vi "Sub Bytes.vi"(2 "Nb":i32=4, 7 "State In":u16[][](array[numeric])=[[125, 216, 135, 144], [71, 71, 164, 177], [128, 52, 170, 55], [161, 141, 234, 198]], 11 "error in":errorcluster) -> (8 "State Out":u16[][](array[numeric]), 15 "error out":errorcluster)   [LabVIEW 2020, in "Library Commun.lvlib" / "Advanced Encryption Standard (AES).lvlib"]
doc: "In the SubBytes step, each byte in the matrix is updated using an 8-bit substitution box, the Rijndael S-box. This operation provides the non-linearity in the cipher. \n\n<inline>"
uses:
  Advanced Encryption Standard (AES).lvlib
panel:
  # "old s= 125,216,135,144,71,71,164,177,128,52,170,55,161,141,234,198"
  # "new s= 255,97,23,96,160,160,73,200,205,24,172,154,50,93,135,180"
  # "255,97,23,96,160,73,200,160,172,154,205,24,        180,50,93,135"
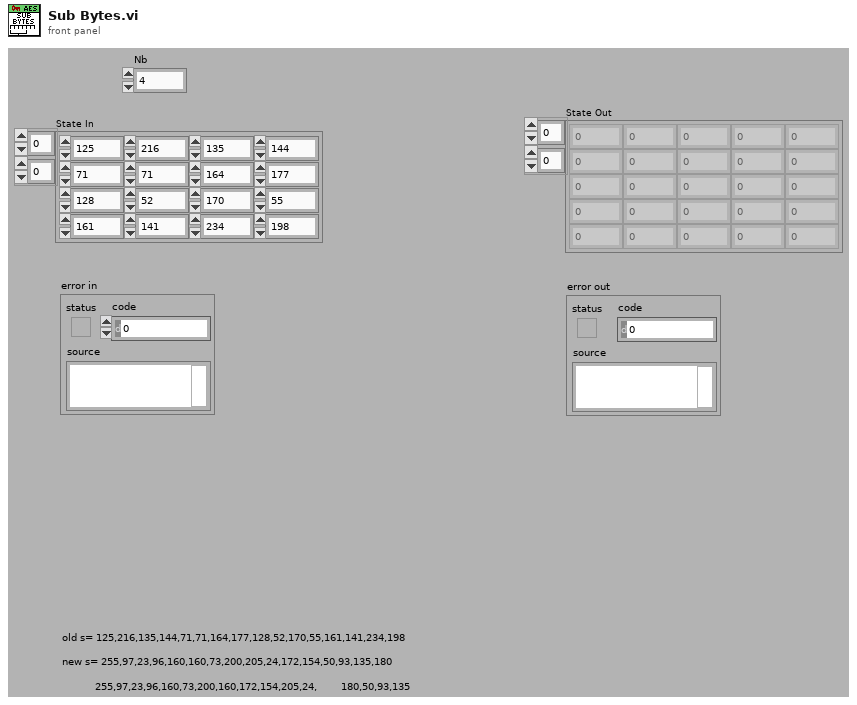
[diagram p1: front panel]
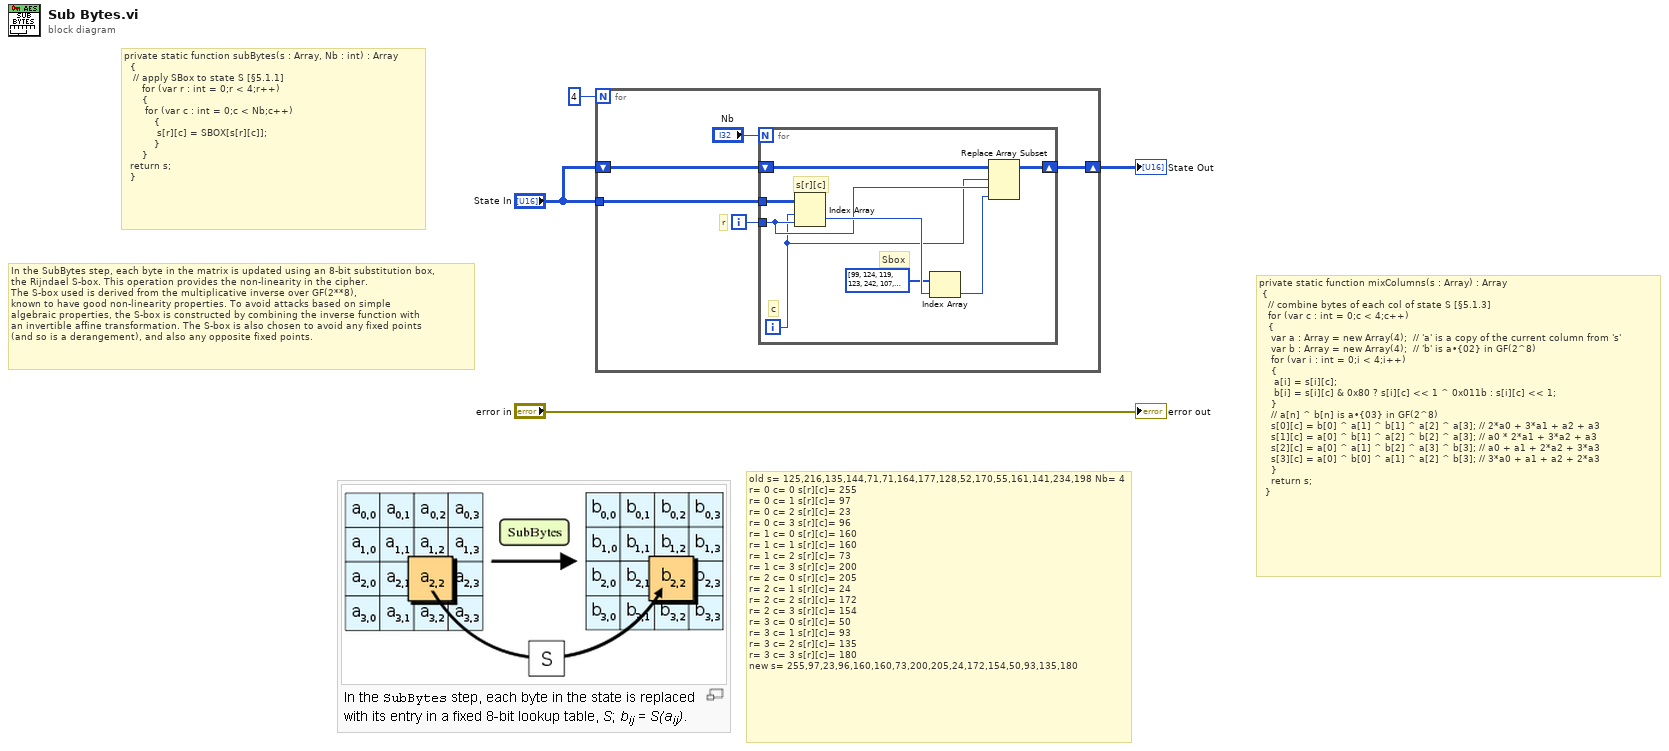
[diagram p0: block diagram]
diagram:
  # "In the SubBytes step, each byte in the matrix is updated using an 8-bit substitution box, \nthe Rijndael S-box. This operation provides the non-linearity in the cipher. \nThe S-box used is derived from the multiplicative inverse over GF(2**8), \nknown to have good non-linearity properties. To avoid attacks based on simple \nalgebraic properties, the S-box is constructed by combining the inverse function with \nan invertible affine transformation. The S-box is also chosen to avoid any fixed points \n(and so is a derangement), and also any opposite fixed points."
  # "old s= 125,216,135,144,71,71,164,177,128,52,170,55,161,141,234,198 Nb= 4\nr= 0 c= 0 s[r][c]= 255\nr= 0 c= 1 s[r][c]= 97\nr= 0 c= 2 s[r][c]= 23\nr= 0 c= 3 s[r][c]= 96\nr= 1 c= 0 s[r][c]= 160\nr= 1 c= 1 s[r][c]= 160\nr= 1 c= 2 s[r][c]= 73\nr= 1 c= 3 s[r][c]= 200\nr= 2 c= 0 s[r][c]= 205\nr= 2 c= 1 s[r][c]= 24\nr= 2 c= 2 s[r][c]= 172\nr= 2 c= 3 s[r][c]= 154\nr= 3 c= 0 s[r][c]= 50\nr= 3 c= 1 s[r][c]= 93\nr= 3 c= 2 s[r][c]= 135\nr= 3 c= 3 s[r][c]= 180\nnew s= 255,97,23,96,160,160,73,200,205,24,172,154,50,93,135,180"
  # "private static function subBytes(s : Array, Nb : int) : Array \n\t\t{    \n\t\t\t// apply SBox to state S [§5.1.1]\n\t\t   \tfor (var r : int = 0;r < 4;r++) \n\t\t   \t{\n\t\t   \t\tfor (var c : int = 0;c < Nb;c++) \n\t\t      \t\t{\n\t\t\t      \t\ts[r][c] = SBOX[s[r][c]];\n\t\t\t      \t}\n   \t\t\t}\n\t\treturn s;\t\t\t\n\t\t}"
  # "private static function mixColumns(s : Array) : Array \n {   \n\t\t\t// combine bytes of each col of state S [§5.1.3]\n\t\t\tfor (var c : int = 0;c < 4;c++) \n\t\t\t{\n\t\t\t\tvar a : Array = new Array(4);  // 'a' is a copy of the current column from 's'\n\t\t\t\tvar b : Array = new Array(4);  // 'b' is a•{02} in GF(2^8)\n\t\t\t\tfor (var i : int = 0;i < 4;i++) \n\t\t\t\t{\n\t\t\t\t\ta[i] = s[i][c];\n\t\t\t\t\tb[i] = s[i][c] & 0x80 ? s[i][c] << 1 ^ 0x011b : s[i][c] << 1;\n\t\t\t\t}\n\t\t\t\t// a[n] ^ b[n] is a•{03} in GF(2^8)\n\t\t\t\ts[0][c] = b[0] ^ a[1] ^ b[1] ^ a[2] ^ a[3]; // 2*a0 + 3*a1 + a2 + a3\n\t\t\t\ts[1][c] = a[0] ^ b[1] ^ a[2] ^ b[2] ^ a[3]; // a0 * 2*a1 + 3*a2 + a3\n\t\t\t\ts[2][c] = a[0] ^ a[1] ^ b[2] ^ a[3] ^ b[3]; // a0 + a1 + 2*a2 + 3*a3\n\t\t\t\ts[3][c] = a[0] ^ b[0] ^ a[1] ^ a[2] ^ b[3]; // 3*a0 + a1 + a2 + 2*a3\n\t\t\t\t}\n\t\t\t\treturn s;\n\t\t}"
  n1 = for {
    N: 4 -> [_]
    tunnel: "State In" -> [w8]
    shift-right: [w5] -> w2
    shift-left: "State In" -> [w7]
    i -> [w9]
    # "r"
    n2 = for {
      N: "Nb" -> [_]
      tunnel: w8 -> [w17]
      tunnel: w9 -> [w14]
      shift-right: [w10] -> w5
      shift-left: w7 -> [w11]
      i -> [w13]
      # "Sbox"
      # "s[r][c]"
      # "c"
      n3 = Index Array(array=w17, index (row)=w13, index (col)=w14) -> (element=w16:u16)
      n4 = Index Array(array=u16[] [99, 124, 119, 123, 242, 107, 111, 197, 48, 1, 103, 43, 254, 215, 171, 118, 202, 130, 201, 125, 250, 89, 71, 240, 173, 212, 162, 175, 156, 164, 114, 192, 183, 253, 147, 38, 54, 63, 247, 204, 52, 165, 229, 241, 113, 216, 49, 21, 4, 199, 35, 195, 24, 150, 5, 154, 7, 18, 128, 226, 235, 39, 178, 117, 9, 131, 44, 26, 27, 110, 90, 160, 82, 59, 214, 179, 41, 227, 47, 132, 83, 209, 0, 237, 32, 252, 177, 91, 106, 203, 190, 57, 74, 76, 88, 207, 208, 239, 170, 251, 67, 77, 51, 133, 69, 249, 2, 127, 80, 60, 159, 168, 81, 163, 64, 143, 146, 157, 56, 245, 188, 182, 218, 33, 16, 255, 243, 210, 205, 12, 19, 236, 95, 151, 68, 23, 196, 167, 126, 61, 100, 93, 25, 115, 96, 129, 79, 220, 34, 42, 144, 136, 70, 238, 184, 20, 222, 94, 11, 219, 224, 50, 58, 10, 73, 6, 36, 92, 194, 211, 172, 98, 145, 149, 228, 121, 231, 200, 55, 109, 141, 213, 78, 169, 108, 86, 244, 234, 101, 122, 174, 8, 186, 120, 37, 46, 28, 166, 180, 198, 232, 221, 116, 31, 75, 189, 139, 138, 112, 62, 181, 102, 72, 3, 246, 14, 97, 53, 87, 185, 134, 193, 29, 158, 225, 248, 152, 17, 105, 217, 142, 148, 155, 30, 135, 233, 206, 85, 40, 223, 140, 161, 137, 13, 191, 230, 66, 104, 65, 153, 45, 15, 176, 84, 187, 22] ("Sbox"), index=w16) -> (element=w15:u16)
      n5 = Replace Array Subset(array=w11, new element=w15, index (row)=w13, index (col)=w14) -> (w10:u16[][])
    }
  }
  "State Out" <- w2
  "error out" <- "error in"
